vi "Problem array.vi"() -> ()   [LabVIEW 2011]
panel:
  out "Result":dbl
  out "Numeric 12":dbl
  out "Numeric 11":dbl
  out "Numeric 10":dbl
  out "Numeric 9":dbl
  out "Numeric 4":dbl
  out "Numeric 3":dbl
  out "Numeric 2":dbl
  out "Numeric":dbl
  in  "Numeric 8":dbl
  in  "Numeric 7":dbl
  in  "Numeric 6":dbl
  in  "Numeric 5":dbl
  in  "Index 4":dbl
  in  "Index 3":dbl
  in  "Index 2":dbl
  in  "Index 1":dbl
  in  "Array":dbl[][](array[numeric])
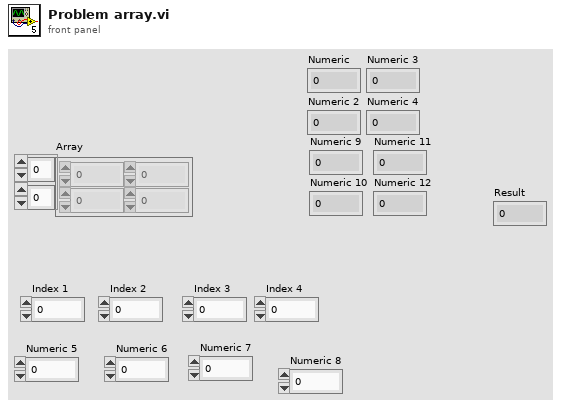
[diagram p1: front panel]
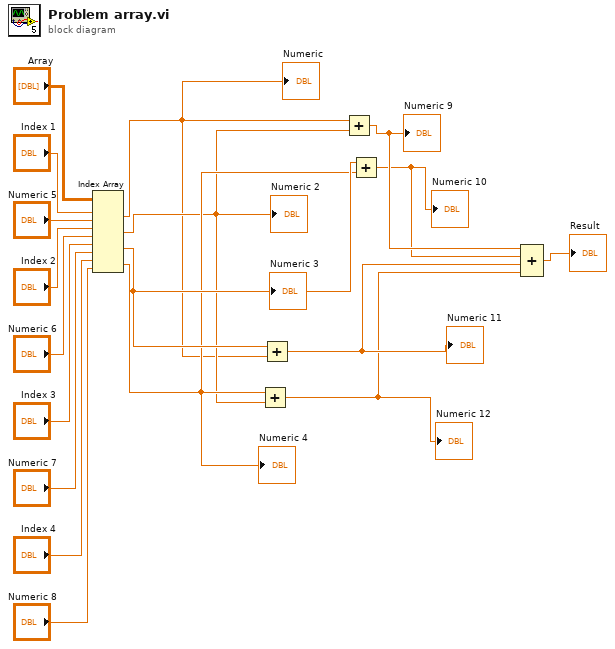
[diagram p0: block diagram]
diagram:
  n1 = Index Array(array="Array", index (row) #1="Index 1", index (col) #1="Numeric 5", index (row) #2="Index 2", index (col) #2="Numeric 6", index (row) #3="Index 3", index (col) #3="Numeric 7", index (row) #4="Index 4", index (col) #4="Numeric 8") -> (element #1=w5:dbl, element #2=w6:dbl, element #3=w8:dbl, element #4=w7:dbl)
  "Numeric" <- w5
  "Numeric 2" <- w6
  "Numeric 3" <- w8
  "Numeric 4" <- w7
  n2 = Add(x=w7, y=w6) -> (x+y=w1:dbl)
  "Numeric 12" <- w1
  n3 = Add(x=w8, y=w5) -> (x+y=w2:dbl)
  "Numeric 11" <- w2
  n4 = Add(x=w5, y=w6) -> (x+y=w4:dbl)
  "Numeric 9" <- w4
  n5 = Add(x=w8, y=w7) -> (x+y=w3:dbl)
  "Numeric 10" <- w3
  n6 = Compound Arithmetic op=ADD(w4, w3, w2, w1) -> (→"Result":dbl)
